vi "Inverter.vi"   [LabVIEW 2016]
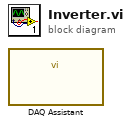
[diagram p0: block diagram]
diagram:
  n1 = call "DAQ Assistant"() -> ()  [unwired: 12 in]
